vi "Post-Register.vi"(8 "error in (no error)":errorcluster, 11 "Instruments in":refnum<class "Instruments.lvclass">) -> (0 "error out":errorcluster, 3 "Instruments out":refnum<class "Instruments.lvclass">)   [LabVIEW 2023, in "Instruments.lvlib" / "Instruments.lvclass"]
doc: "<b>Post Register</b>\nThis routine is implemented in <b>Post Launch Initialize</b> after the actor has registered for events.\n\nIt's intended to provide a means of performing actions immediately before the actor state engine is entered."
uses:
  Library/Instruments.lvclass
  Library/Instruments.lvclass/Instruments.ctl
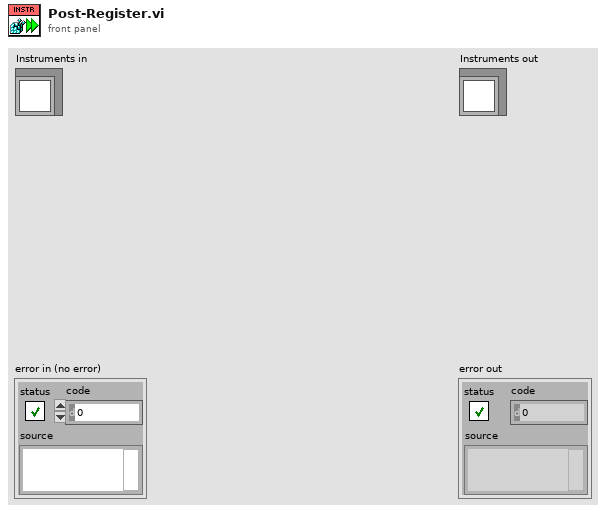
[diagram p1: front panel]
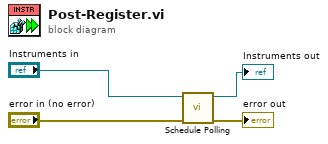
[diagram p0: block diagram]
diagram:
  n1 = call "Schedule Polling.vi"("error in (no error)"="error in (no error)", "Instruments in"="Instruments in") -> ("error out"=→"error out":errorcluster, "Instruments out"=→"Instruments out":refnum<class "Instruments.lvclass">)  [unwired: 8 in]
